vi "sliderOpen.vi"() -> ()   [LabVIEW 2017]
uses:
  globalDevices.vi
  <vilib>/Instr/_visa.llb/VISA Configure Serial Port (Instr).vi
panel:
  out "success":bool
  out "read buffer":string
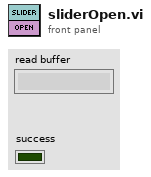
[diagram p1: front panel]
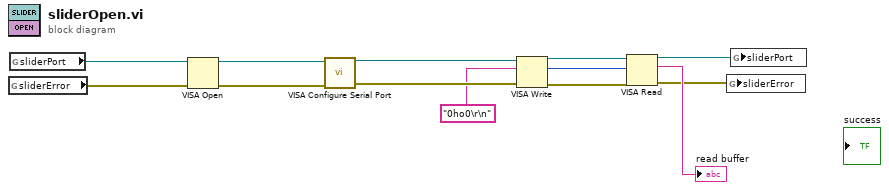
[diagram p0: block diagram]
diagram:
  n1 = global read "globalDevices.vi" "sliderError"() -> (w13:errorcluster)
  n2 = global read "globalDevices.vi" "sliderPort"() -> (w12:refnum<visa-resource-name>)
  n3 = VISA Open(error in (no error)=w13, VISA resource name=w12) -> (VISA resource name=w11:refnum<visa-resource-name>, error out=w10:errorcluster)  [unwired: 3 in]
  n4 = call-poly "VISA Configure Serial Port"("VISA resource name"=w11, "error in (no error)"=w10) -> ("VISA resource name out"=w3:refnum<visa-resource-name>, "error out"=w2:errorcluster)  [unwired: 12 in]
  n5 = VISA Write(VISA resource name=w3, write buffer="0ho0\r\n", error in (no error)=w2) -> (VISA resource name out=w8:refnum<visa-resource-name>, return count=w9:u32, error out=w7:errorcluster)
  n6 = VISA Read(VISA resource name=w8, byte count=w9, error in (no error)=w7) -> (VISA resource name out=w5:refnum<visa-resource-name>, read buffer=→"read buffer":string, error out=w4:errorcluster)  [unwired: 1 out]
  n7 = global write "globalDevices.vi" "sliderError"(w4) -> ()
  n8 = global write "globalDevices.vi" "sliderPort"(w5) -> ()
